vi "Cannon Process.vi"   [LabVIEW 2013]
uses:
  Cannon Global.vi
types:
  T1 = typedef "WPI_RelayValue.ctl" = enum16{"Off", "On", "Forward", "Reverse"}
  T2 = cluster{"Angle":dbl, "Clutch MS":bool, "Ball MS":bool, "Clutch ":T1, "LeFireatwill":bool, "Arm":bool, "Armed":bool, "Fire!":bool, "Bottom MS":bool, "Motor VBus":dbl}
  T3 = cluster{"Angle":dbl, "Clutch MS":bool, "Ball MS":bool, "Motor VBus":dbl, "Clutch ":T1, "LeFireatwill":bool, "Arm":bool, "Armed":bool, "Fire!":bool, "Bottom MS":bool}
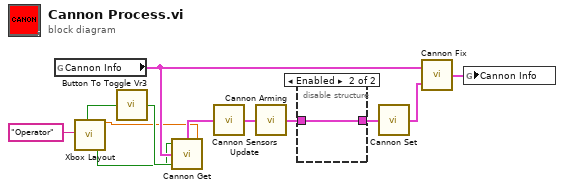
[diagram p0: block diagram]
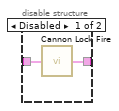
[diagram p2: hidden frame]
diagram:
  n1 = global read "Cannon Global.vi" "Cannon Info"() -> (w7:T2)
  n2 = call "Xbox Layout.vi"("Joystick Name"="Operator") -> ("Left Button"=w5:bool, "Y"=w2:bool, "Left Stick Y"=w1:dbl)  [unwired: 3 in, 13 out]
  n3 = call "Button To Toggle Vr3.vi"("InValue"=w5) -> ("Result"=w3:bool)
  n4 = call "Cannon Get.vi"("Motor VBus"=w1, "Arm?"=w3, "Cannon Info"=w7, "Shoot"=w2) -> ("Cannon Info 2"=w6:T2)
  n5 = call "Cannon Sensors Update.vi"("Cannon Info In"=w6) -> ("Cannon Info  Out"=w9:T2)
  n6 = call "Cannon Arming.vi"("Cannon Info In"=w9) -> ("Cannon Info Out"=w12:T2)
  n7 = disable-structure shown="Enabled" {
    disable-tunnel: w12 -> [w14 w15]
    disable-tunnel: [w13 w15] -> w8
    frame Disabled {
      n8 = call "Cannon Lock Fire.vi"("Cannon Info In"=w14) -> ("Cannon Info Out"=w13:T3)
    }
    frame Enabled {
    }
  }
  n9 = call "Cannon Set.vi"("Cannon Info In"=w8) -> ("Cannon Info Out"=w11:T2)
  n10 = call "Cannon Fix.vi"("Cannon Info Modified"=w11, "Cannon Info Original"=w7) -> ("Cannon Info Fixed"=w10:T2)
  n11 = global write "Cannon Global.vi" "Cannon Info"(w10) -> ()
